vi "Task ID.vi"(8 "error in (no error)":errorcluster, 11 "VolatusConfigManager in":refnum<class "VolatusConfigManager.lvclass">) -> (0 "error out":errorcluster, 2 "Task ID":string, 3 "VolatusConfigManager out":refnum<class "VolatusConfigManager.lvclass">)   [LabVIEW 2020, in "Volatus.lvlib" / "VolatusConfigManager.lvclass"]
uses:
  VolatusConfigManager.lvclass
  VolatusConfigManager.lvclass/VolatusConfigManager.ctl
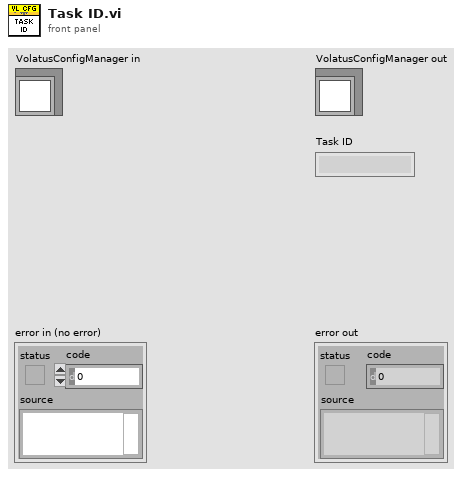
[diagram p1: front panel]
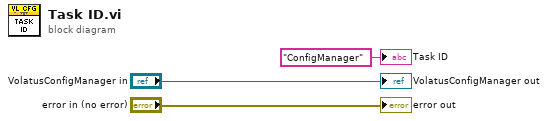
[diagram p0: block diagram]
diagram:
  "error out" <- "error in (no error)"
  "VolatusConfigManager out" <- "VolatusConfigManager in"
  "Task ID" <- "ConfigManager" ("Task ID")
